vi "读取excel配置信息.vi"(8 "error in (no error)":errorcluster, 10 "测试参数":string="频率显示", 11 "report in":refnum<class "NI_report.lvclass">) -> (0 "error out":errorcluster, 2 "配置信息":string[][](array[string]), 3 "report out":refnum<class "NI_report.lvclass">)   [LabVIEW 2015]
uses:
  <vilib>/Utility/NIReport.llb/NI_report.lvclass
  <vilib>/addons/_office/excel.llb/Excel Get Data ([str]).vi
  <vilib>/Utility/NIReport.llb/Excel/NI_Excel.lvclass
  <vilib>/addons/_office/NI_ReportGenerationToolkit.lvlib
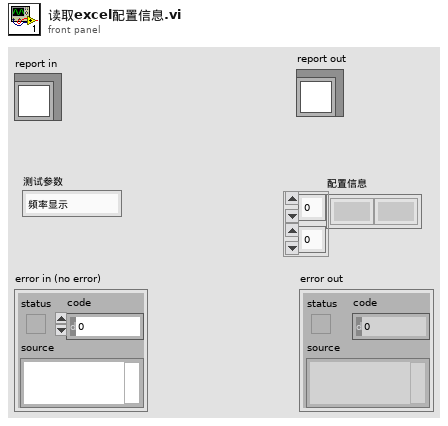
[diagram p1: front panel]
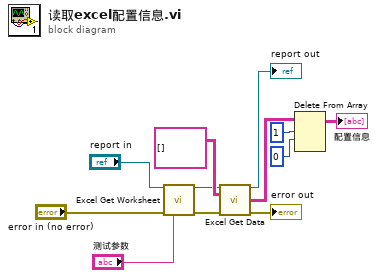
[diagram p0: block diagram]
diagram:
  n1 = call <vilib>:"Excel Get Worksheet.vi"("report in"="report in", "error in (no error)"="error in (no error)", "name (\"\")"="测试参数") -> ("report out"=w10:refnum<class "NI_report.lvclass">, "error out"=w11:errorcluster)  [unwired: 11 in]
  n2 = call-poly <vilib>:"Excel Get Data.vi"("report in"=w10, "data type"=string[][] [], "error in (no error)"=w11) -> ("report out"=→"report out":refnum<class "NI_report.lvclass">, "data"=w6:string[][], "error out"=→"error out":errorcluster)  [unwired: 10 in]
  n3 = Delete From Array(array=w6, length=1 ("禁用的索引 (列)"), index (row)=0 ("索引 (行)")) -> (array with subset deleted=→"配置信息":string[][])  [unwired: 1 in, 1 out]
